vi "VI2.vi"() -> ()   [LabVIEW 2010]
panel:
  in  "ARMAZEM_PEGAR":bool
  in  "ESTEIRA_PEGAR":bool
  in  "Elevar_Z":dbl min=0.0 max=2.0
  out "YD3":dbl
  out "YD2":dbl
  out "YD1":dbl
  out "YD0":dbl
  in  "Coordenada_Y":dbl min=0.0 max=2.0
  out "Z_Pos_Ok":bool
  out "Y_Pos_Ok":bool
  out "X_Pos_Ok":bool
  out "Z_Home_Ok":bool
  out "Y_Home_Ok":bool
  out "X_Home_Ok":bool
  in  "Z_CTRG":bool
  in  "Y_CTRG":bool
  in  "X_CTRG":bool
  in  "Z_HOME":bool
  in  "Y_HOME":bool
  in  "X_HOME":bool
  in  "Start":bool
  in  "Confirmação da posição":bool
  out "ZD3":dbl
  out "ZD2":dbl
  out "ZD1":dbl
  out "ZD0":dbl
  out "XD3":dbl
  out "XD2":dbl
  out "XD1":dbl
  out "XD0":dbl
  in  "Coordenada_Z":dbl min=0.0 max=10.0
  in  "Coordenada_X":dbl min=0.0 max=6.0
  out "Esteira 4":bool
  out "Esteira 3":bool
  out "Esteira 2":bool
  out "Esteira 1":bool
  in  "Eletroválvula 4":bool
  in  "Eletroválvula 3":bool
  in  "Eletroválvula 2":bool
  in  "Eletroválvula 1":bool
  out "Sensor 4":bool
  out "Sensor 3":bool
  out "Sensor 2":bool
  out "Sensor 1":bool
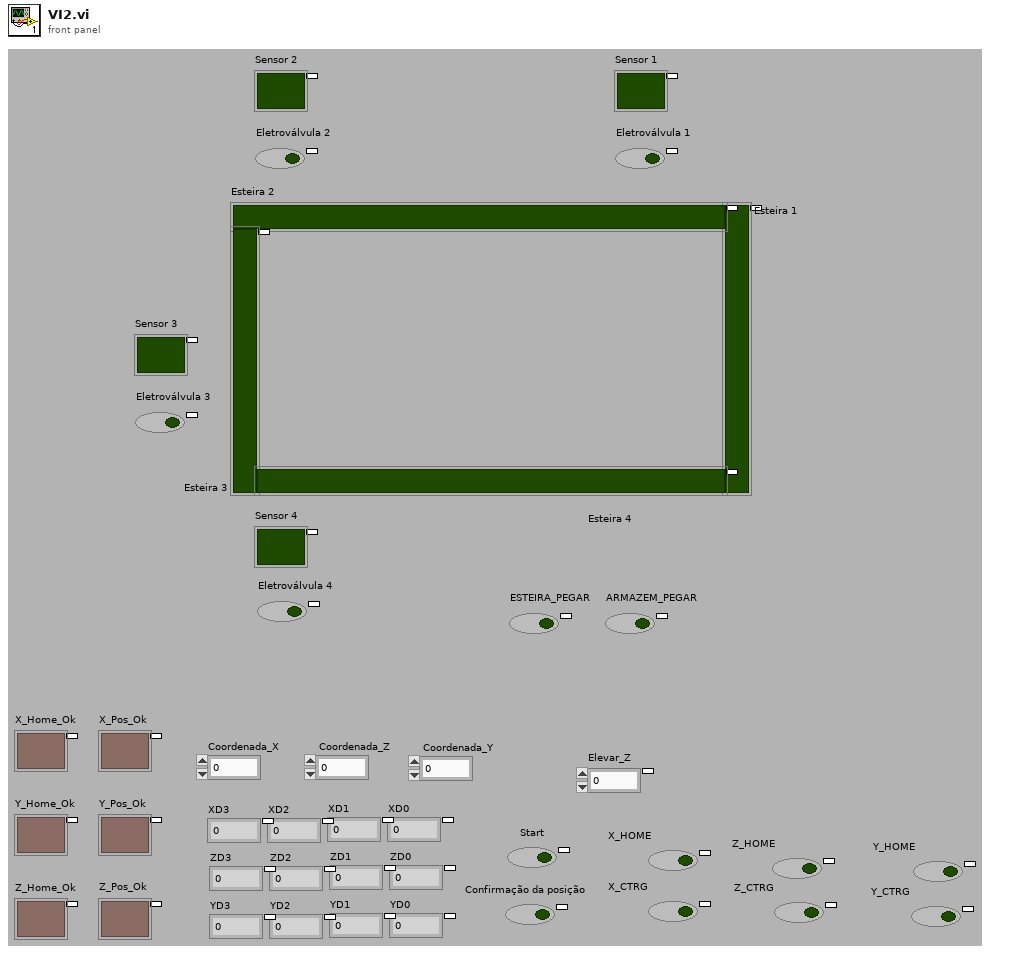
[diagram p1: front panel]
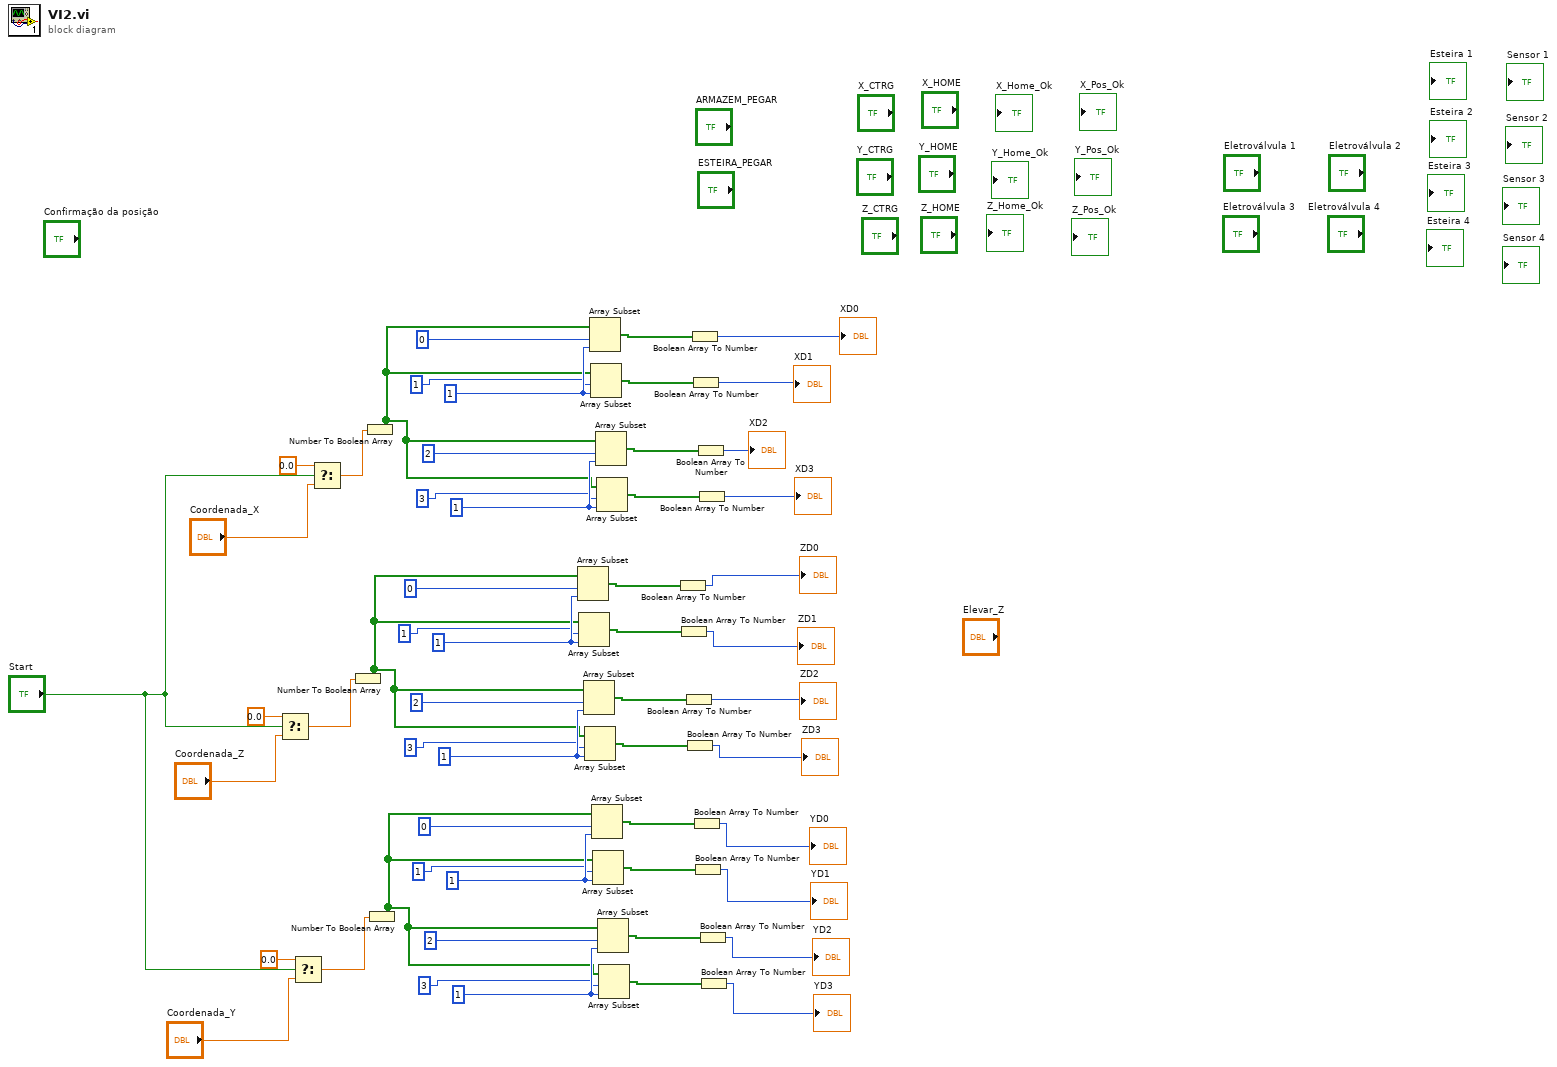
[diagram p0: block diagram]
diagram:
  w17 = 1 ("index")
  w22 = 1 ("index")
  w32 = 1 ("index")
  w37 = 1 ("index")
  w47 = 1 ("index")
  w52 = 1 ("index")
  n1 = Select(t=0.0, s="Start", f="Coordenada_Z") -> (s? t:f=w3:dbl)
  n2 = Select(t=0.0, s="Start", f="Coordenada_Y") -> (s? t:f=w1:dbl)
  n3 = Select(t=0.0, s="Start", f="Coordenada_X") -> (s? t:f=w5:dbl)
  n4 = Number To Boolean Array(number=w3) -> (Boolean array=w30:bool[])
  n5 = Number To Boolean Array(number=w5) -> (Boolean array=w45:bool[])
  n6 = Number To Boolean Array(number=w1) -> (Boolean array=w15:bool[])
  n7 = Array Subset(array=w30, index=0, length=w37) -> (w40:bool[])
  n8 = Array Subset(array=w30, index=1, length=w37) -> (w38:bool[])
  n9 = Array Subset(array=w30, index=2, length=w32) -> (w35:bool[])
  n10 = Array Subset(array=w30, index=3, length=w32) -> (w33:bool[])
  n11 = Array Subset(array=w45, index=0, length=w52) -> (w55:bool[])
  n12 = Array Subset(array=w45, index=1, length=w52) -> (w53:bool[])
  n13 = Array Subset(array=w15, index=0, length=w22) -> (w25:bool[])
  n14 = Array Subset(array=w15, index=1, length=w22) -> (w23:bool[])
  n15 = Array Subset(array=w45, index=2, length=w47) -> (w50:bool[])
  n16 = Array Subset(array=w45, index=3, length=w47) -> (w48:bool[])
  n17 = Array Subset(array=w15, index=2, length=w17) -> (w20:bool[])
  n18 = Array Subset(array=w15, index=3, length=w17) -> (w18:bool[])
  n19 = Boolean Array To Number(Boolean array=w40) -> (number=→"ZD0":u32)
  n20 = Boolean Array To Number(Boolean array=w38) -> (number=→"ZD1":u32)
  n21 = Boolean Array To Number(Boolean array=w35) -> (number=→"ZD2":u32)
  n22 = Boolean Array To Number(Boolean array=w33) -> (number=→"ZD3":u32)
  n23 = Boolean Array To Number(Boolean array=w55) -> (number=→"XD0":u32)
  n24 = Boolean Array To Number(Boolean array=w53) -> (number=→"XD1":u32)
  n25 = Boolean Array To Number(Boolean array=w25) -> (number=→"YD0":u32)
  n26 = Boolean Array To Number(Boolean array=w23) -> (number=→"YD1":u32)
  n27 = Boolean Array To Number(Boolean array=w50) -> (number=→"XD2":u32)
  n28 = Boolean Array To Number(Boolean array=w48) -> (number=→"XD3":u32)
  n29 = Boolean Array To Number(Boolean array=w20) -> (number=→"YD2":u32)
  n30 = Boolean Array To Number(Boolean array=w18) -> (number=→"YD3":u32)
